vi "Launcher.vi"   [LabVIEW 2020]
uses:
  [V] Tester Parent/[V] Tester Parent/[V] Tester Parent.lvclass
  C:/Program Files (x86)/National Instruments/LabVIEW 2020/vi.lib/ActorFramework/Actor/Actor.lvclass
  <vilib>/ActorFramework/Actor/Actor.lvclass
panel:
  # "Launcher"
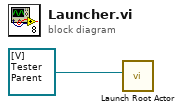
[diagram p0: block diagram]
diagram:
  n1 = call <vilib>:"Launch Root Actor.vi"("Actor"=refnum<class "[V] Tester Parent.lvclass"> refnum ("[V] Tester Parent.lvlib:[V] Tester Parent.lvclass")) -> ()  [unwired: 9 in, 2 out]
